vi "Auto-Cycle.vi"(8 "error in (no error)":errorcluster, 11 "AD4212C in":refnum<class "AD4212C.lvclass">) -> (0 "error out":errorcluster, 3 "AD4212C out":refnum<class "AD4212C.lvclass">)   [LabVIEW 2014, in "AD4212C.lvlib" / "AD4212C.lvclass"]
uses:
  AD4212C.lvclass
  AD4212C.lvclass/AD4212C.ctl
  <vilib>/Utility/error.llb/Error Cluster From Error Code.vi
  <vilib>/ErrorRing/Error Ring.xnode
  DriverMasterAsync/builds/DriverMasterAsync.lvlibp/Modules/HAL/DriverMasterAsync/DriverMasterAsyncClass/DriverMasterAsync.lvclass
  API/AD4212C Lib.lvlib
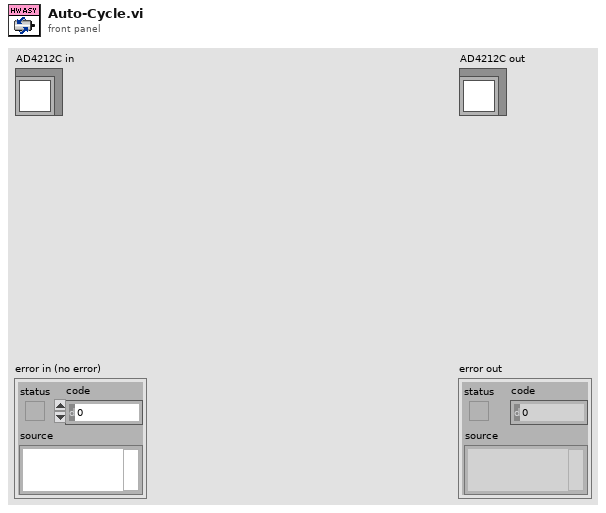
[diagram p1: front panel]
types:
  T1 = typedef "AD4212C Lib.lvlib/Connection Data.ctl" = cluster{"Conection Data":refnum<visa-resource-name>}
  T2 = typedef "DriverMasterAsync.lvlibp/WINFAS 2 Data Queue.lvlib/Async Acquisition Data Cluster.ctl" = cluster{"Data":sgl[]}
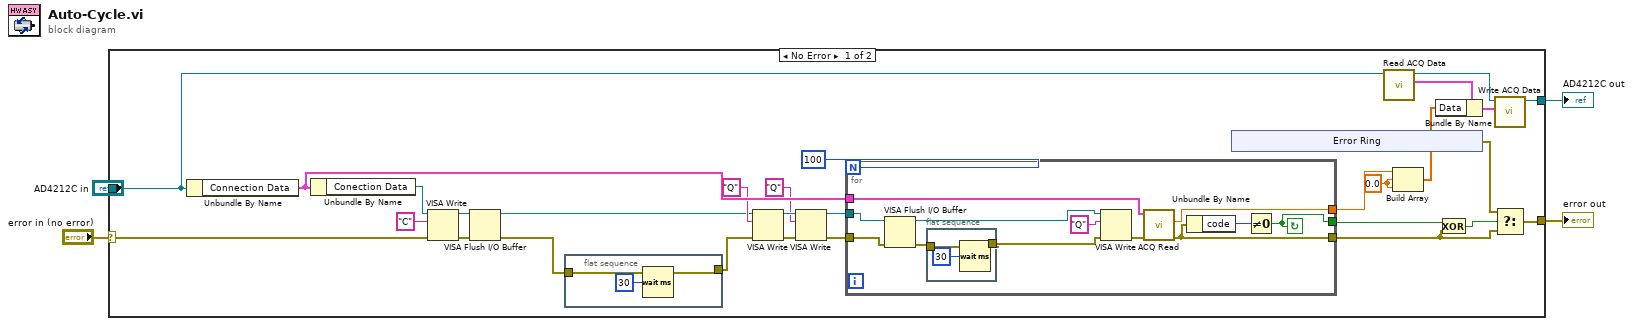
[diagram p0: block diagram]
diagram:
  n1 = case shown="No Error" "error in (no error)" {
    selector: "error in (no error)" -> [w26 w56]
    tunnel: [w17 w56] -> w3
    tunnel: [w33 w55] -> w1
    tunnel: "AD4212C in" -> [w30 w55]
    frame No Error {
      w23 = sgl 0.0 ("default value 1")
      n2 = Unbundle By Name(w30) -> ("Connection Data"=w21:T1)
      n3 = Unbundle By Name(w21) -> ("Conection Data"=w28:refnum<visa-resource-name>)
      n4 = VISA Write(VISA resource name=w28, write buffer="C", error in (no error)=w26) -> (VISA resource name out=w25:refnum<visa-resource-name>, error out=w24:errorcluster)  [unwired: 1 out]
      n5 = VISA Flush I/O Buffer(VISA resource name=w25, error in (no error)=w24) -> (VISA resource name out=w10:refnum<visa-resource-name>, error out=w6:errorcluster)  [unwired: 1 in]
      n6 = flat-sequence {
        tunnel: w6 -> [w35]
        tunnel: [w35] -> w5
        frame #0 {
          n7 = Wait (ms)(milliseconds to wait=u32 30) -> ()  [unwired: 1 out]
        }
      }
      n8 = VISA Write(VISA resource name=w10, write buffer="Q", error in (no error)=w5) -> (VISA resource name out=w15:refnum<visa-resource-name>, error out=w16:errorcluster)  [unwired: 1 out]
      n9 = VISA Write(VISA resource name=w15, write buffer="Q", error in (no error)=w16) -> (VISA resource name out=w12:refnum<visa-resource-name>, error out=w11:errorcluster)  [unwired: 1 out]
      n10 = for {
        N: 100 -> [_]
        tunnel: w12 -> [w44]
        tunnel: w21 -> [w51]
        tunnel: [w50] -> w20
        tunnel: w11 -> [w45]
        tunnel: [w48] -> w9
        tunnel: [w46] -> w8
        stop <- w46 continue-if-true
        n11 = VISA Flush I/O Buffer(VISA resource name=w44, error in (no error)=w45) -> (VISA resource name out=w41:refnum<visa-resource-name>, error out=w43:errorcluster)  [unwired: 1 in]
        n12 = flat-sequence {
          tunnel: w43 -> [w54]
          tunnel: [w54] -> w42
          frame #0 {
            n13 = Wait (ms)(milliseconds to wait=u32 30) -> ()  [unwired: 1 out]
          }
        }
        n14 = VISA Write(VISA resource name=w41, write buffer="Q", error in (no error)=w42) -> (error out=w49:errorcluster)  [unwired: 2 out]
        n15 = call "ACQ Read.vi"("error in (no error)"=w49, "VISA resource name In"=w51) -> ("error out"=w48:errorcluster, "Value"=w50:sgl)  [unwired: 7 in, 1 out]
        n16 = Unbundle By Name(w48) -> ("code"=w47:i32)
        n17 = Not Equal To 0?(x=w47) -> (x != 0?=w46:bool)
      }
      n18 = xnode "Error Ring"() -> ("error out"=w18:errorcluster)
      n19 = call "Read ACQ Data.vi"("DriverMasterAsync in"=w30) -> ("ACQ Data"=w32:T2, "DriverMasterAsync out"=w29:refnum<class "AD4212C.lvclass">)  [unwired: 8 in, 1 out]
      n20 = Build Array(w20, w23, w23) -> (w22:sgl[])
      n21 = Bundle By Name(cluster=w32, "Data"=w22) -> (w31:T2)
      n22 = Exclusive Or(1:w9, 2:w8) -> (0:w7:bool)
      n23 = call "Write ACQ Data.vi"("ACQ Data"=w31, "DriverMasterAsync in"=w29) -> ("DriverMasterAsync out"=w33:refnum<class "AD4212C.lvclass">)  [unwired: 8 in, 1 out]
      n24 = Select(t=w18, s=w7, f=w9) -> (s? t:f=w17:errorcluster)
    }
    frame Error {
    }
  }
  "error out" <- w3
  "AD4212C out" <- w1
